vi "Open scan SEQ.vi"(0 "dup path":path, 1 "End wavelength":dbl, 5 "Crop top":i32, 7 "delim":string=",", 9 "Crop bottom":dbl, 11 "Start wavelength":dbl) -> (3 "wavelengths":sgl[](array[numeric]), 14 "Intensities":sgl[](array[numeric]))   [LabVIEW 2014]
uses:
  <vilib>/Utility/file.llb/Read From Spreadsheet File (DBL).vi
  Subs/Global 1.vi
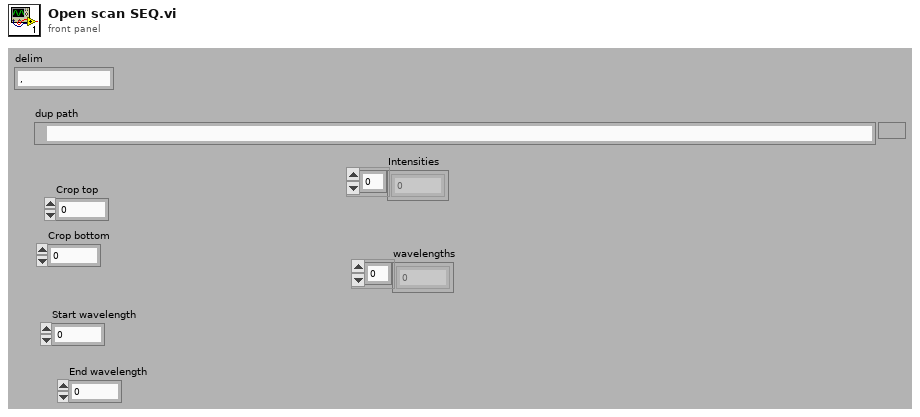
[diagram p1: front panel]
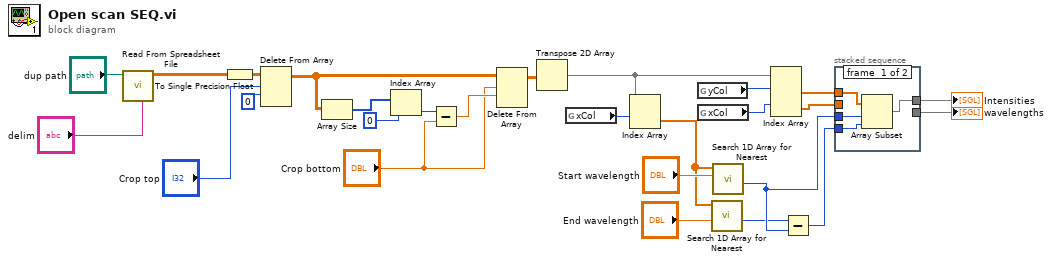
[diagram p0: block diagram]
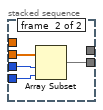
[diagram p2: hidden frame]
diagram:
  n1 = call-poly <vilib>:"Read From Spreadsheet File.vi"("delimiter (\\t)"="delim", "file path (dialog if empty)"="dup path") -> ("all rows"=w25:dbl[][])  [unwired: 5 in, 4 out]
  n2 = To Single Precision Float(number=w25) -> (single precision float=w26:sgl[][])
  n3 = Delete From Array(array=w26, length="Crop top", index (row)=0) -> (array with subset deleted=w13:sgl[][])  [unwired: 1 in, 1 out]
  n4 = Array Size(array=w13) -> (size(s)=w17:i32[])
  n5 = Index Array(array=w17, index=0) -> (element=w14:i32)
  n6 = Subtract(x=w14, y="Crop bottom") -> (x-y=w15:dbl)
  n7 = Delete From Array(array=w13, length="Crop bottom", index (row)=w15) -> (array with subset deleted=w18:sgl[][])  [unwired: 1 in, 1 out]
  n8 = Transpose 2D Array(2D array=w18) -> (transposed array=w27:sgl[][])
  n9 = global read "Global 1.vi" "xCol"() -> (w3:i32)
  n10 = Index Array(array=w27, index (row)=w3) -> (element=w7:sgl[])  [unwired: 1 in]
  n11 = global read "Global 1.vi" "yCol"() -> (w1:i32)
  n12 = global read "Global 1.vi" "xCol"() -> (w2:i32)
  n13 = call "Search 1D Array for Nearest.vi"("desired element"="End wavelength", "1D Array"=w7) -> ("closest index"=w6:i32)  [unwired: 8 in, 1 out]
  n14 = call "Search 1D Array for Nearest.vi"("desired element"="Start wavelength", "1D Array"=w7) -> ("closest index"=w9:i32)  [unwired: 8 in, 1 out]
  n15 = Index Array(array=w27, index (row) #1=w1, index (row) #2=w2) -> (element #1=w20:sgl[], element #2=w21:sgl[])  [unwired: 2 in]
  n16 = Subtract(x=w6, y=w9) -> (x-y=w24:i32)
  n17 = stacked-sequence {
    tunnel: w20 -> [w31 _]
    tunnel: w9 -> [w30 w34]
    tunnel: w24 -> [w29 w33]
    tunnel: w21 -> [_ w35]
    tunnel: [_ w32] -> w22
    tunnel: [w28 _] -> w23
    frame #0 {
      n18 = Array Subset(array=w31, index=w30, length=w29) -> (w28:sgl[])
    }
    frame #1 {
      n19 = Array Subset(array=w35, index=w34, length=w33) -> (w32:sgl[])
    }
  }
  "Intensities" <- w23
  "wavelengths" <- w22
